vi "FPGA DC SERVO.vi"() -> ()   [LabVIEW 2015]
uses:
  <vilib>/rvi/Emulation/niFpgaGetClockAttributes.vi
  <vilib>/rvi/Emulation/niFpgaSctlEmulationGetInTimedLoop.vi
  <vilib>/rvi/Emulation/niFpgaEmulationReportErrorSimple.vi
  <vilib>/rvi/Emulation/niFpgaCriticalErrorInLSC.vi
  <instrlib>/Parallax Standard Servo/FPGA/NI_Robotics_Parallax Standard Servo (FPGA).lvlib
panel:
  in  "servo_0_ccw angle":fxp<+/-,32,4>
  in  "servo_0_ccw offset":fxp<+/-,32,4>
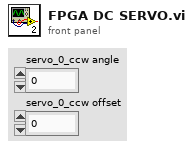
[diagram p1: front panel]
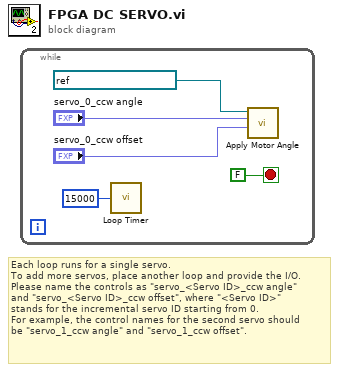
[diagram p0: block diagram]
diagram:
  # "Each loop runs for a single servo.\nTo add more servos, place another loop and provide the I/O.\nPlease name the controls as \"servo_<Servo ID>_ccw angle\"\nand \"servo_<Servo ID>_ccw offset\", where \"<Servo ID>\"\nstands for the incremental servo ID starting from 0.\nFor example, the control names for the second servo should\nbe \"servo_1_ccw angle\" and \"servo_1_ccw offset\"."
  n1 = while "Sensor Servo Motor Control Loop" {
    stop <- FALSE stop-if-true
    n2 = call "Loop Timer"("Count(uSec)"=u32 15000) -> ()  [unwired: 1 out]
    n3 = call <instrlib>:"Apply Motor Angle.vi"("ccw angle offset (rad)"="servo_0_ccw offset", "ccw angle (rad)"="servo_0_ccw angle", "digital output line"=refnum<k21> "ConnectorC/DIO1" ("Servo")) -> ()  [unwired: 9 in]
  }
